vi "checkStatus.vi"(8 "error in (no error)":errorcluster, 10 "stop":bool, 11 "NetworkWinX32 in":refnum<class "NetworkWinX32.lvclass">) -> (0 "error out":errorcluster, 2 "stopped?":bool, 3 "NetworkWinX32 out":refnum<class "NetworkWinX32.lvclass">)   [LabVIEW 2011, in "Hardware.lvlib" / "HWControllers.lvlib" / "NetworkWinX32.lvclass"]
uses:
  NetworkWinX32.lvclass
  NetworkWinX32.lvclass/NetworkWinX32.ctl
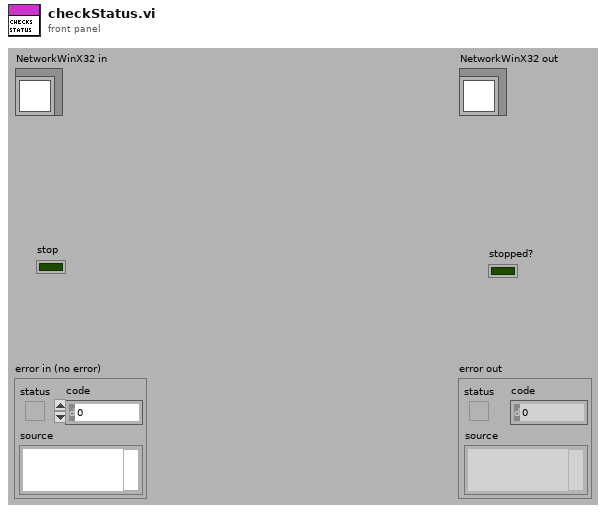
[diagram p1: front panel]
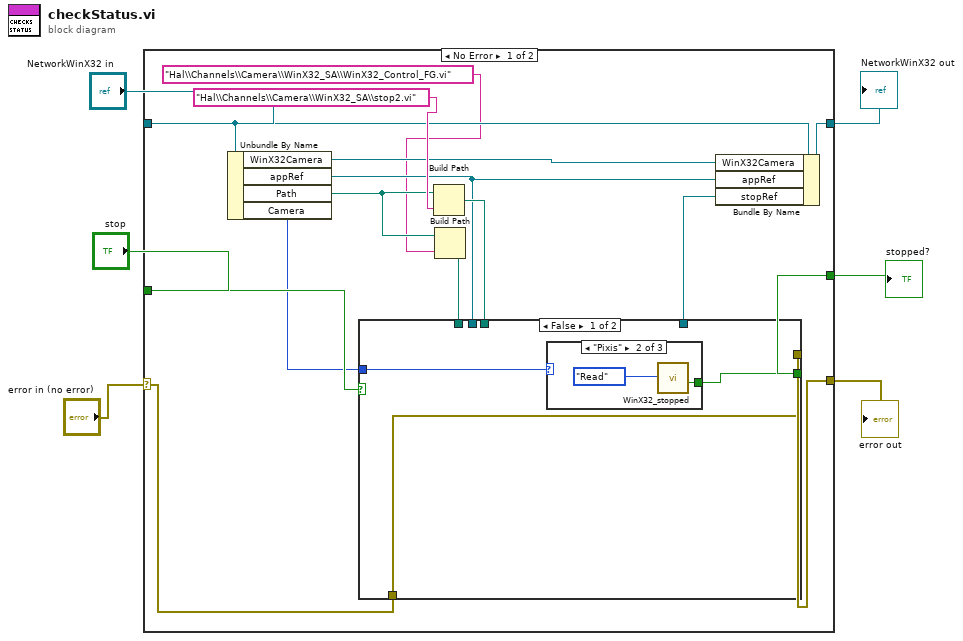
[diagram p0: block diagram]
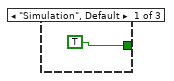
[diagram p2: hidden frame]
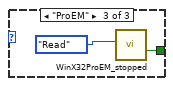
[diagram p3: hidden frame]
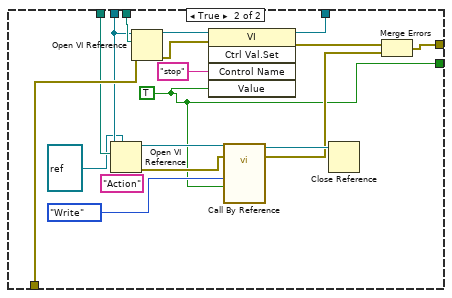
[diagram p4: hidden frame]
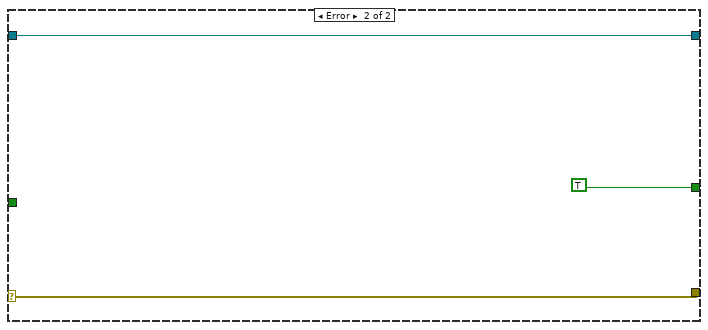
[diagram p5: hidden frame]
diagram:
  n1 = case shown="No Error" "error in (no error)" {
    selector: "error in (no error)" -> [w19 w48]
    tunnel: [w14 w48] -> w2
    tunnel: "NetworkWinX32 in" -> [w16 w49]
    tunnel: [w15 w49] -> w5
    tunnel: "stop" -> [w13 _]
    tunnel: [w18 TRUE] -> w1
    frame No Error {
      n2 = Unbundle By Name(w16) -> ("WinX32Camera"=w12:refnum<class "WinX32Camera.lvclass">, "appRef"=w17:refnum<vi>, "Path"=w9:path, "Camera"=w10:enum16{"Simulation", "Pixis", "ProEM"})
      n3 = Build Path(base path=w9, name or relative path="Hal\\Channels\\Camera\\WinX32_SA\\stop2.vi") -> (appended path=w20:path)
      n4 = Build Path(base path=w9, name or relative path="Hal\\Channels\\Camera\\WinX32_SA\\WinX32_Control_FG.vi") -> (appended path=w7:path)
      n5 = case shown="False" w13 {
        tunnel: w20 -> [_ w46]
        tunnel: w19 -> [w24 w45]
        tunnel: [w23 w30] -> w18
        tunnel: w17 -> [_ w41]
        tunnel: [w24 w38] -> w14
        tunnel: [_ w42] -> w11
        tunnel: w10 -> [w22 _]
        tunnel: w7 -> [_ w40]
        frame False {
          n6 = case shown="\"Pixis\"" w22 {
            tunnel: [TRUE w27 w28] -> w23
            frame "Simulation", Default {
            }
            frame "Pixis" {
              n7 = call "WinX32_stopped.vi"("Action"=enum16{"Write", "Read"}."Read") -> ("stopped"=w27:bool)  [unwired: 10 in]
            }
            frame "ProEM" {
              n8 = call "WinX32ProEM_stopped.vi"("Action"=enum16{"Write", "Read"}."Read") -> ("stopped"=w28:bool)  [unwired: 10 in]
            }
          }
        }
        frame True {
          (unwired) "Action"
          w30 = TRUE
          n9 = Open VI Reference(type specifier VI Refnum (for type only)=refnum<vi> refnum ("reference"), application reference (local)=w41, vi path=w40) -> (vi reference=w34:refnum<vi>, error out=w36:errorcluster)  [unwired: 3 in]
          n10 = Open VI Reference(application reference (local)=w41, vi path=w46, error in (no error)=w45) -> (vi reference=w43:refnum<vi>, error out=w44:errorcluster)  [unwired: 3 in]
          n11 = invoke class="VI" method="Ctrl Val.Set"(reference=w43, error in=w44, "Control Name"="stop", "Value"=w30) -> (reference out=w42:refnum<vi>, error out=w37:errorcluster)  [unwired: 1 in, 3 out]
          n12 = call-by-ref "?"(reference=w34, error in=w36, "stop"=w30, "Action"=enum16{"Write", "Read"}."Write") -> (reference out=w33:refnum<vi>, error out=w32:errorcluster)  [unwired: 9 in, 1 out]
          n13 = Close Reference(reference=w33) -> ()  [unwired: 1 in, 1 out]
          n14 = Merge Errors(w37, w32) -> (w38:errorcluster)
        }
      }
      n15 = Bundle By Name(cluster=w16, "WinX32Camera"=w12, "appRef"=w17, "stopRef"=w11) -> (w15:refnum<class "NetworkWinX32.lvclass">)
    }
    frame Error {
    }
  }
  "error out" <- w2
  "NetworkWinX32 out" <- w5
  "stopped?" <- w1
